vi "Motion Plot.vi"() -> ()   [LabVIEW 2017]
panel:
  out "Dist max (mm)":dbl
  out "V max (mm/s)":dbl
  in  "Motion Parameters":T1={"Decel Time (s)"=0.0, "Accel Time (s)"=0.0, "Total Time (s)"=0.0, "Max Accel (mm/s^2)"=0.0, "Max Decel (mm/s^2)"=0.0, "Time step (s)"=0.01} {"Time step (s)" min=0.001}
  out "Displacement":dbl[](graph)
  out "Velocity":dbl[](graph)
  out "Acceleration":dbl[](graph)
  # "Use 0.01s"
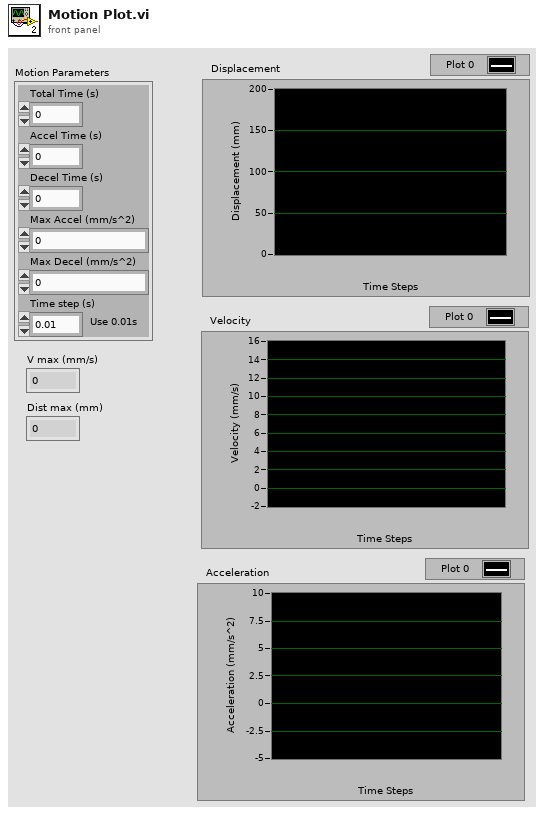
[diagram p1: front panel]
types:
  T1 = cluster{"Decel Time (s)":dbl, "Accel Time (s)":dbl, "Total Time (s)":dbl, "Max Accel (mm/s^2)":dbl, "Max Decel (mm/s^2)":dbl, "Time step (s)":dbl}
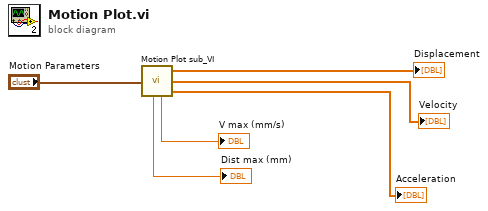
[diagram p0: block diagram]
diagram:
  n1 = call "Motion Plot sub_VI.vi"("Motion Parameters"="Motion Parameters") -> ("Dist max (mm)"=→"Dist max (mm)":dbl, "Displacement"=→"Displacement":dbl[], "Velocity"=→"Velocity":dbl[], "V max (mm/s)"=→"V max (mm/s)":dbl, "Acceleration"=→"Acceleration":dbl[])  [unwired: 4 in]
